vi "CalcSummaryUncertainties_TempTest.vi"(8 "error in (no error)":errorcluster, 10 "Limits":dbl[][][](array[numeric]), 11 "Uncertainties":dbl[][][](array[numeric]) format="%.6f") -> (0 "error out":errorcluster, 3 "PFI":string[][][](array[string]))   [LabVIEW 2014]
uses:
  typedef/PMUConfig_TempTests.ctl
panel:
  in  "Tab Control":enum32{"Uncertainties", "Limits", "PFI"}(tab)
  # "V+ TVE"
  # "I+ TVE"
  # "VA TVE"
  # "VB TVE"
  # "VC TVE"
  # "IA TVE"
  # "IB TVE"
  # "IC TVE"
  # "Freq Hz"
  # "ROCOF HZ/s"
  # "FreqRng"
  # "MagRng"
  # "Harmonics"
  # "Out-of-Band"
  # "Amplitude Mod"
  # "Phase Mod"
  # "FreqRamp +"
  # "FreqRamp -"
  # "VA TVE"
  # "VB TVE"
  # "VC TVE"
  # "V+ TVE"
  # "IA TVE"
  # "IB TVE"
  # "IC TVE"
  # "I+ TVE"
  # "FE"
  # "RFE"
  # "FreqRng"
  # "MagRng"
  # "Harm"
  # "OOB"
  # "Phase Mod"
  # "Ampl Mod"
  # "Freq Ramp +"
  # "Freq Ramp -"
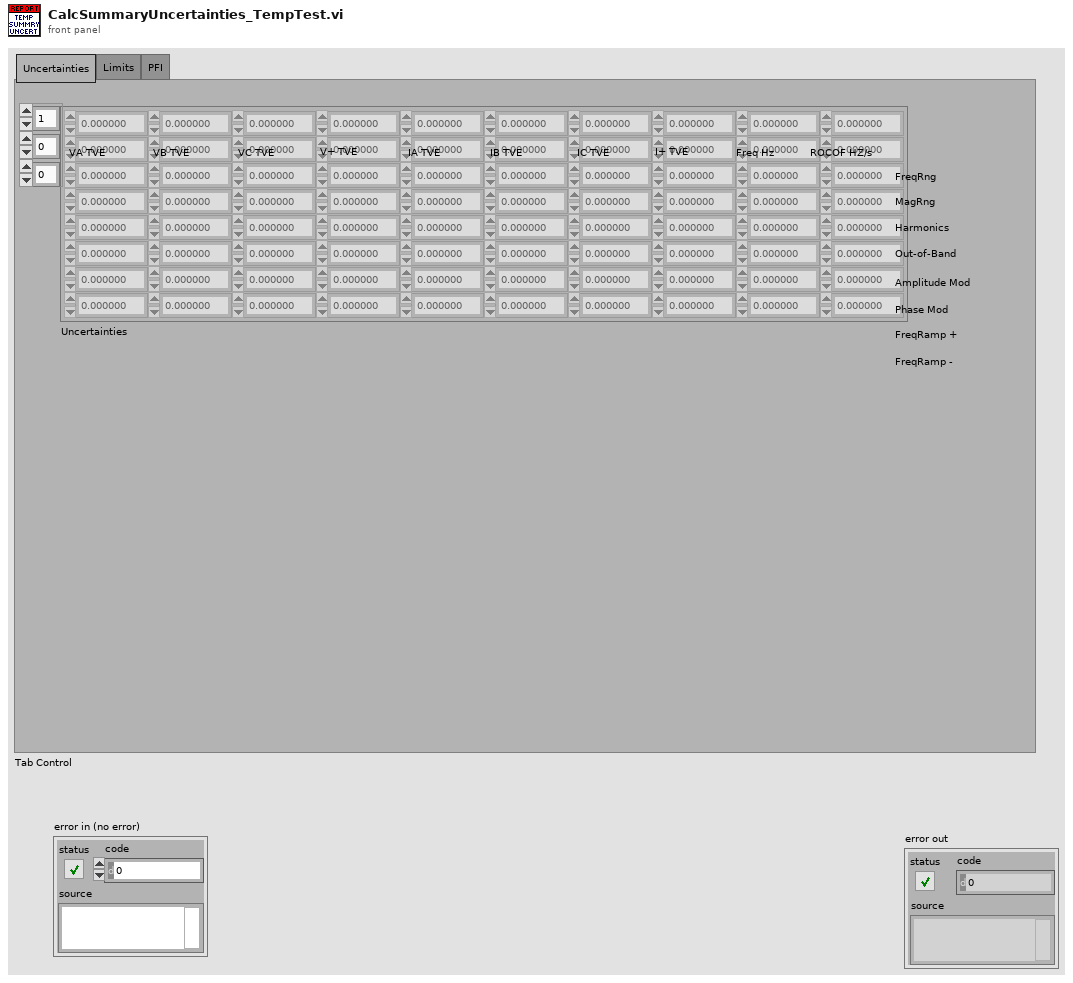
[diagram p1: front panel]
types:
  T1 = typedef "PMUConfig_TempTests.ctl" = cluster{"Class":string, "Fs":dbl, "F0":dbl, "Temp":string}
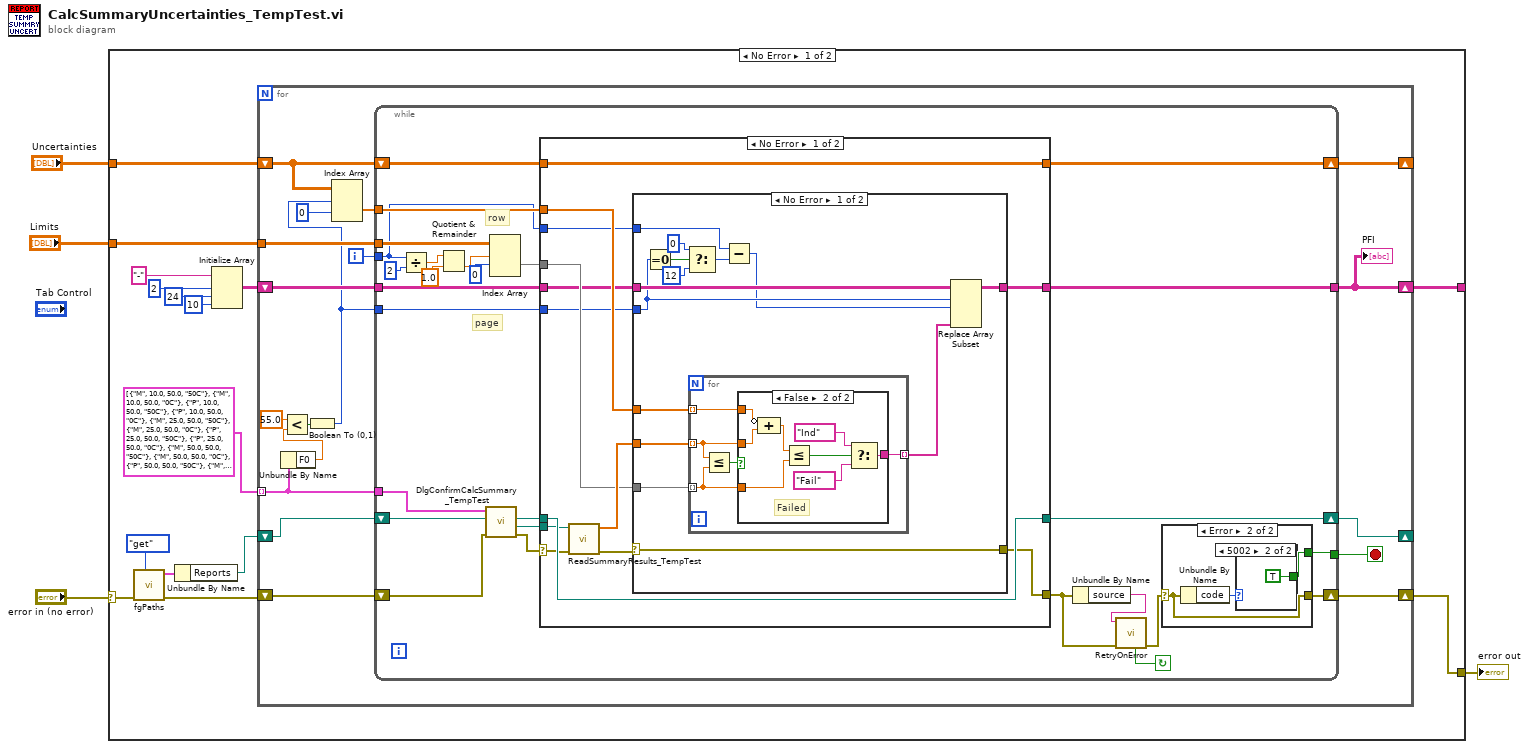
[diagram p0: block diagram]
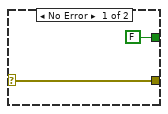
[diagram p2: hidden frame]
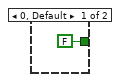
[diagram p3: hidden frame]
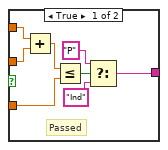
[diagram p4: hidden frame]
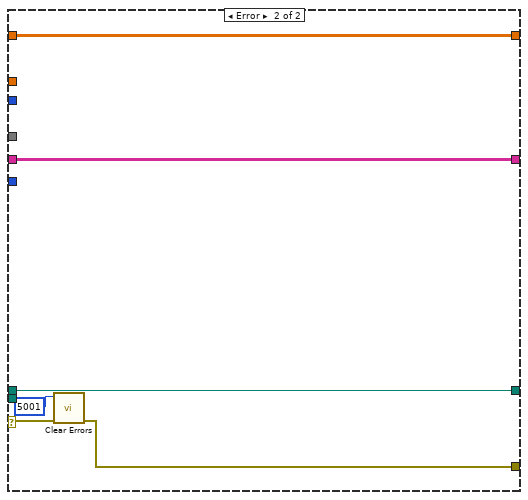
[diagram p6: hidden frame]
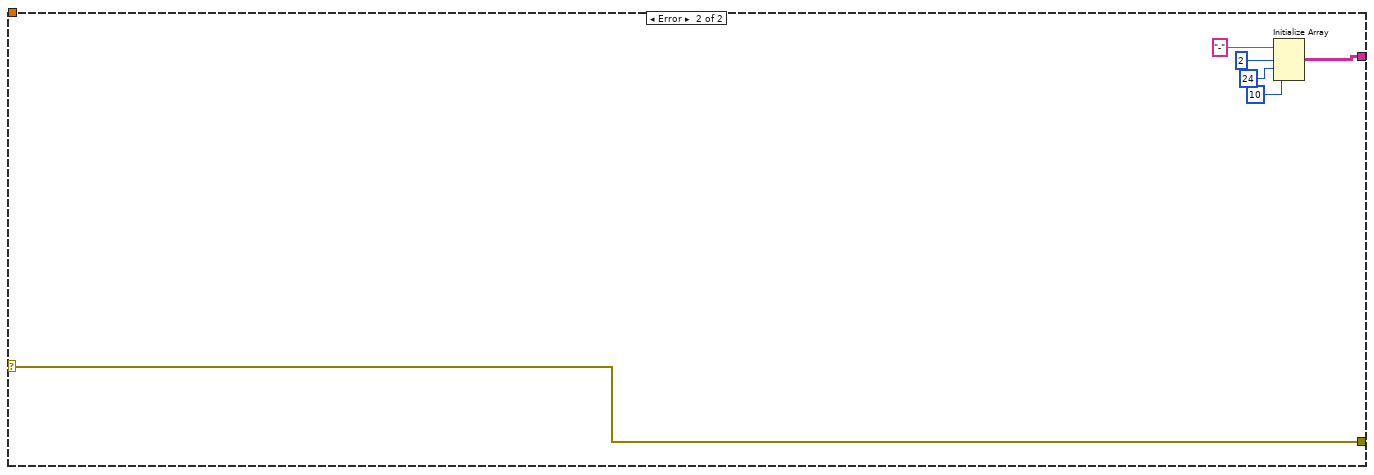
[diagram p7: hidden frame]
diagram:
  n1 = case shown="No Error" "error in (no error)" {
    selector: "error in (no error)" -> [w14 w133]
    tunnel: [w18 w133] -> w3
    tunnel: "Uncertainties" -> [w17 _]
    tunnel: "Limits" -> [w16 _]
    tunnel: [w5 w128] -> _
    frame No Error {
      n2 = call "fgPaths.vi"("cmd"=enum16{"init", "set", "get"}."get", "error in (no error)"=w14) -> ("error out"=w13:errorcluster, "clPaths"=w15:cluster{"Templates":path, "Reports":path})  [unwired: 8 in]
      n3 = Unbundle By Name(w15) -> ("Reports"=w12:path)
      n4 = Initialize Array("-", 2 ("dimension size"), 24 ("dimension size"), 10 ("dimension size")) -> (w6:string[][][])
      n5 = for {
        tunnel: T1[] [{"Class"="M", "Fs"=10.0, "F0"=50.0, "Temp"="50C"}, {"Class"="M", "Fs"=10.0, "F0"=50.0, "Temp"="0C"}, {"Class"="P", "Fs"=10.0, "F0"=50.0, "Temp"="50C"}, {"Class"="P", "Fs"=10.0, "F0"=50.0, "Temp"="0C"}, {"Class"="M", "Fs"=25.0, "F0"=50.0, "Temp"="50C"}, {"Class"="M", "Fs"=25.0, "F0"=50.0, "Temp"="0C"}, {"Class"="P", "Fs"=25.0, "F0"=50.0, "Temp"="50C"}, {"Class"="P", "Fs"=25.0, "F0"=50.0, "Temp"="0C"}, {"Class"="M", "Fs"=50.0, "F0"=50.0, "Temp"="50C"}, {"Class"="M", "Fs"=50.0, "F0"=50.0, "Temp"="0C"}, {"Class"="P", "Fs"=50.0, "F0"=50.0, "Temp"="50C"}, {"Class"="M", "Fs"=50.0, "F0"=50.0, "Temp"="0C"}, {"Class"="M", "Fs"=10.0, "F0"=60.0, "Temp"="50C"}, {"Class"="M", "Fs"=10.0, "F0"=60.0, "Temp"="0C"}, {"Class"="P", "Fs"=10.0, "F0"=60.0, "Temp"="50C"}, {"Class"="P", "Fs"=10.0, "F0"=60.0, "Temp"="0C"}, {"Class"="M", "Fs"=12.0, "F0"=60.0, "Temp"="50C"}, {"Class"="M", "Fs"=12.0, "F0"=60.0, "Temp"="0C"}, {"Class"="P", "Fs"=12.0, "F0"=60.0, "Temp"="50C"}, {"Class"="P", "Fs"=12.0, "F0"=60.0, "Temp"="0C"}, {"Class"="M", "Fs"=15.0, "F0"=60.0, "Temp"="50C"}, {"Class"="M", "Fs"=15.0, "F0"=60.0, "Temp"="0C"}, {"Class"="P", "Fs"=15.0, "F0"=60.0, "Temp"="50C"}, {"Class"="P", "Fs"=15.0, "F0"=60.0, "Temp"="0C"}, {"Class"="M", "Fs"=20.0, "F0"=60.0, "Temp"="50C"}, {"Class"="M", "Fs"=20.0, "F0"=60.0, "Temp"="0C"}, {"Class"="P", "Fs"=20.0, "F0"=60.0, "Temp"="50C"}, {"Class"="P", "Fs"=20.0, "F0"=60.0, "Temp"="0C"}, {"Class"="M", "Fs"=30.0, "F0"=60.0, "Temp"="50C"}, {"Class"="M", "Fs"=30.0, "F0"=60.0, "Temp"="0C"}, {"Class"="P", "Fs"=30.0, "F0"=60.0, "Temp"="50C"}, {"Class"="P", "Fs"=30.0, "F0"=60.0, "Temp"="0C"}, {"Class"="M", "Fs"=60.0, "F0"=60.0, "Temp"="50C"}, {"Class"="M", "Fs"=60.0, "F0"=60.0, "Temp"="0C"}, {"Class"="P", "Fs"=60.0, "F0"=60.0, "Temp"="50C"}, {"Class"="P", "Fs"=60.0, "F0"=60.0, "Temp"="0C"}] -> [w30] mode=indexing
        shift-right: [w34] -> w18
        shift-left: w13 -> [w36]
        shift-right: [w33] -> _
        shift-left: w17 -> [w31]
        shift-right: [w32] -> _
        shift-left: w12 -> [w37]
        tunnel: w16 -> [w25]
        shift-right: [w20] -> w5
        shift-left: w6 -> [w23]
        i -> [w24]
        stop <- w35 stop-if-true
        n6 = Unbundle By Name(w30) -> ("F0"=w29:dbl)
        n7 = Less?(x=55.0, y=w29) -> (x < y?=w27:bool)
        n8 = Boolean To (0,1)(Boolean=w27) -> (0, 1=w22:i16)
        n9 = Index Array(array=w31, index (dim 0)=w22, index (dim 1)=0 ("disabled index (row)")) -> (element=w26:dbl[])  [unwired: 1 in]
        n10 = while {
          tunnel: w30 -> [w64]
          tunnel: [w50] -> w35
          shift-right: [w56] -> w32
          shift-left: w37 -> [w63]
          shift-right: [w51] -> w34
          shift-left: w36 -> [w62]
          shift-right: [w59] -> w33
          shift-left: w31 -> [w60]
          tunnel: w26 -> [w49]
          tunnel: w25 -> [w48]
          tunnel: w24 -> [w42]
          tunnel: w23 -> [w46]
          tunnel: w22 -> [w45]
          tunnel: [w43] -> w20
          stop <- w55 continue-if-true
          # "row"
          # "page"
          n11 = Divide(x=w42, y=2) -> (x/y=w41:dbl)
          n12 = Quotient & Remainder(x=w41, y=1.0) -> (floor(x/y)=w38:dbl)  [unwired: 1 out]
          n13 = call "DlgConfirmCalcSummary_TempTest.vi"("error in (no error)"=w62, "Path"=w63, "PMUConfig 2"=w64) -> ("error out"=w61:errorcluster, "Summary Data Excel File"=w58:path, "Path"=w57:path)  [unwired: 5 in, 1 out]
          n14 = Index Array(array=w48, index (dim 0)=w38, index (dim 1)=0 ("disabled index (row)")) -> (element=w47:dbl[])  [unwired: 1 in]
          n15 = case shown="No Error" w61 {
            selector: w61 -> [w83 w127]
            tunnel: [w81 w126] -> w54
            tunnel: w60 -> [w78 w124]
            tunnel: [w78 w124] -> w59
            tunnel: w58 -> [w82 _]
            tunnel: w57 -> [w84 w123]
            tunnel: [w84 w123] -> w56
            tunnel: w49 -> [w79 _]
            tunnel: w47 -> [w77 _]
            tunnel: w46 -> [w75 w122]
            tunnel: w45 -> [w74 _]
            tunnel: w42 -> [w73 _]
            tunnel: [w72 w122] -> w43
            frame No Error {
              n16 = call "ReadSummaryResults_TempTest.vi"("error in (no error)"=w83, "Path"=w82) -> ("error out"=w76:errorcluster, "Results"=w80:dbl[])  [unwired: 8 in]
              n17 = case shown="No Error" w76 {
                selector: w76 -> [w98 w121]
                tunnel: [w98 w121] -> w81
                tunnel: w77 -> [w95 _]
                tunnel: w79 -> [w96 _]
                tunnel: w80 -> [w97 _]
                tunnel: w75 -> [w89 w120]
                tunnel: w74 -> [w87 _]
                tunnel: w73 -> [w90 _]
                tunnel: [w85 w120] -> w72
                frame No Error {
                  n18 = Equal To 0?(x=w87) -> (x = 0?=w94:bool)
                  n19 = Select(t=0, s=w94, f=12) -> (s? t:f=w91:i32)
                  n20 = for {
                    tunnel: w95 -> [w101] mode=indexing
                    tunnel: w97 -> [w100] mode=indexing
                    tunnel: w96 -> [w102] mode=indexing
                    tunnel: [w99] -> w88 mode=indexing
                    n21 = Less Or Equal?(x=w100, y=w101) -> (x <= y?=w103:bool)
                    n22 = case shown="False" w103 {
                      tunnel: w102 -> [w111 w119]
                      tunnel: w101 -> [w108 w116]
                      tunnel: w100 -> [w110 w118]
                      tunnel: [w104 w112] -> w99
                      frame True {
                        # "Passed"
                        n23 = Add(x=w111, y=w110) -> (x+y=w109:dbl)
                        n24 = Less Or Equal?(x=w109, y=w108) -> (x <= y?=w107:bool)
                        n25 = Select(t="P", s=w107, f="Ind") -> (s? t:f=w104:string)
                      }
                      frame False {
                        # "Failed"
                        n26 = Compound Arithmetic op=ADD(invert w119, w118) -> (w117:dbl)
                        n27 = Less Or Equal?(x=w117, y=w116) -> (x <= y?=w115:bool)
                        n28 = Select(t="Ind", s=w115, f="Fail") -> (s? t:f=w112:string)
                      }
                    }
                  }
                  n29 = Subtract(x=w90, y=w91) -> (x-y=w86:i32)
                  n30 = Replace Array Subset(array=w89, new element=w88, index (dim 0)=w87, index (dim 1)=w86) -> (w85:string[][][])  [unwired: 1 in]
                }
                frame Error {
                }
              }
            }
            frame Error {
              n31 = call <vilib>:"Clear Errors.vi"("error in (no error)"=w127, "specific error code to clear (0: all)"=5001) -> ("error out"=w126:errorcluster)  [unwired: 4 in, 1 out]
            }
          }
          n32 = Unbundle By Name(w54) -> ("source"=w53:string)
          n33 = call "RetryOnError.vi"("error in (no error)"=w54, "Error Msg"=w53) -> ("error out"=w52:errorcluster, "Retry"=w55:bool)  [unwired: 8 in]
          n34 = case shown="Error" w52 {
            selector: w52 -> [w66 w67]
            tunnel: [w66 w67] -> w51
            tunnel: [FALSE w68] -> w50
            frame No Error {
            }
            frame Error {
              n35 = Unbundle By Name(w67) -> ("code"=w69:i32)
              n36 = case shown="5002" w69 {
                tunnel: [FALSE TRUE] -> w68
                frame 0, Default {
                }
                frame 5002 {
                }
              }
            }
          }
        }
        "PFI" <- w20
      }
    }
    frame Error {
      n37 = Initialize Array("-", 2 ("dimension size"), 24 ("dimension size"), 10 ("dimension size")) -> (w128:string[][][])
    }
  }
  "error out" <- w3
